vi "SimulatoreStep.vi"() -> ()   [LabVIEW 2019]
doc: "Simulatore Step dei Test:\n\n1. Seleziona la postazione con la data di partenza (opzionale)\n2. Seleziona il Test che vuoi eseguire\n3. Avvia la simulazione e verifica il successo degli Step"
uses:
  ByteGSAPIBase.lvclass
  TypeDef/StepSimulationInfo.ctl
  TypeDef/SimulatoreStates.ctl
  TypeDef/Step.ctl
  TypeDef/Asset.ctl
  TypeDef/Test.ctl
  <vilib>/numeric/Random Number (Range) U64.vi
  <vilib>/numeric/sub_Random U32.vi
panel:
  out "Step Info List":T1[](array[typedef])=[{"info"="Descrizione:\nMeasure T0\nMIN - MAX: 23 - 18", "Value"=0.0, "Outcome"="", "Tempo"=0.0, "id"=0.0}, {"info"="Descrizione:\nSet Nominsl Torque\nMIN - MAX: 1 - -1", "Value"=0.0, "Outcome"="", "Tempo"=0.0, "id"=0.0}, {"info"="Descrizione:\nVibrazione X,Y,Z\nMIN - MAX: 0 - 0", "Value"=0.0, "Outcome"="", "Tempo"=0.0, "id"=0.0}, {"info"="Descrizione:\nPlace Motor on the bench. Plug wires on terminal block.\nMIN - MAX: 0 - 0", "Value"=0.0, "Outcome"="", "Tempo"=0.0, "id"=0.0}, {"info"="Descrizione:\nMeasure R01\nMIN - MAX: 0 - 0", "Value"=0.0, "Outcome"="", "Tempo"=0.0, "id"=0.0}, {"info"="Descrizione:\nMeasure R02\nMIN - MAX: 0 - 0", "Value"=0.0, "Outcome"="", "Tempo"=0.0, "id"=0.0}]
  in  "Step simulation":bool
  out "Infos":string
  in  "Inizia Test":bool
  in  "Seleziona Test":i32(ring) items=["Test Endurance"=36, "Test su Statore H100 dia 65"=31, "Test su Statore H100 dia 65"=29, "Test Endurance"=34, "Test su Statore H100 dia 65"=30, "Effettuare prova sul banco Labview su campione ABC"=40, "Test su Statore H100 dia 65"=28, "Test su Statore H100 dia 65"=32, "Richiesta prova 1"=7, "Test Endurance"=35, "Richiesta prova 1"=5, "Richiesta prova 1"=6, "Test su Statore H100 dia 65"=27, "Test doppio carico per freni 50Nm/12rpm"=24]
  in  "ByteGSAPIBase in":refnum<class "ByteGSAPIBase.lvclass">
  in  "Exit":bool
  in  "Home":bool
  in  "Ottieni Test Per Postazione":bool
  in  "Data Partenza":timestamp format="%<%x>T"
  in  "Postazione":enum16{"POST 1"}(ring)
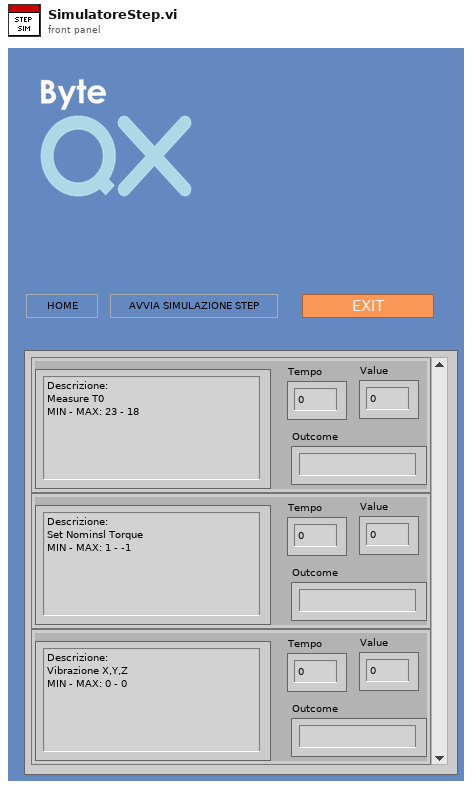
[diagram p1: front panel]
types:
  T1 = typedef "StepSimulationInfo.ctl" = cluster{"info":string, "Value":dbl, "Outcome":string, "Tempo":dbl, "id":dbl}
  T2 = typedef "SimulatoreStates.ctl" = enum16{"Initialize", "Idle", "GetLimsTestsForBench", "GetLimsTestSteps", "Simulation Start"}
  T3 = typedef "ByteGSWebAPI.lvlib/ByteGSAPIBase.lvclass/Test.ctl" = cluster{"titolo":string, "descrizione":string, "statoprova":string, "assets":T4[], "id":i32, "data_apertura_prova":timestamp}
  T4 = typedef "ByteGSWebAPI.lvlib/ByteGSAPIBase.lvclass/Asset.ctl" = cluster{"descrizione":string, "slug":string, "id":i32}
  T5 = typedef "ByteGSWebAPI.lvlib/ByteGSAPIBase.lvclass/Step.ctl" = cluster{"id":i32, "descrizione":string, "prova":string, "assets":T4[], "criterio_accettazione":string, "valore_criterio_accettazione_max":dbl, "valore_criterio_accettazione_min":dbl, "udm_criterio_accettazione":string, "duration_prova":string, "udm_duration_prova":string, "valore_prova":dbl, "outcome":string, "ordine":i32, "user":i32, "link_automation":string, "instruction_automation":string, "data_completamento_checklist":timestamp}
  T6 = cluster{"ByteGSAPIBase in":refnum<class "ByteGSAPIBase.lvclass">, "Array dei Test":T3[], "Steps Array":T5[], "Step Info List":T1[], "index":i32, "Previus":T2, "Infos":string}
  T7 = cluster{"Postazione":refnum<vi>, "Data Partenza":refnum<vi>, "Ottieni Test Per Postazione":refnum<vi>, "Infos":refnum<vi>, "Inizia Test":refnum<vi>, "Seleziona Test":refnum<vi>, "Step Info List":refnum<vi>, "Step simulation":refnum<vi>, "Cluster":refnum<vi>}
  T8 = cluster{"Postazione":enum16{"POST 1"}, "Data Partenza":timestamp, "Seleziona Test":i32}
  T9 = typedef "UpdateLimsTestStepData.ctl" = cluster{"duration_prova":string, "udm_duration_prova":string, "valore_prova":dbl, "outcome":string, "data_completamento_checklist":timestamp, "link_automation":string, "instruction_automation":string}
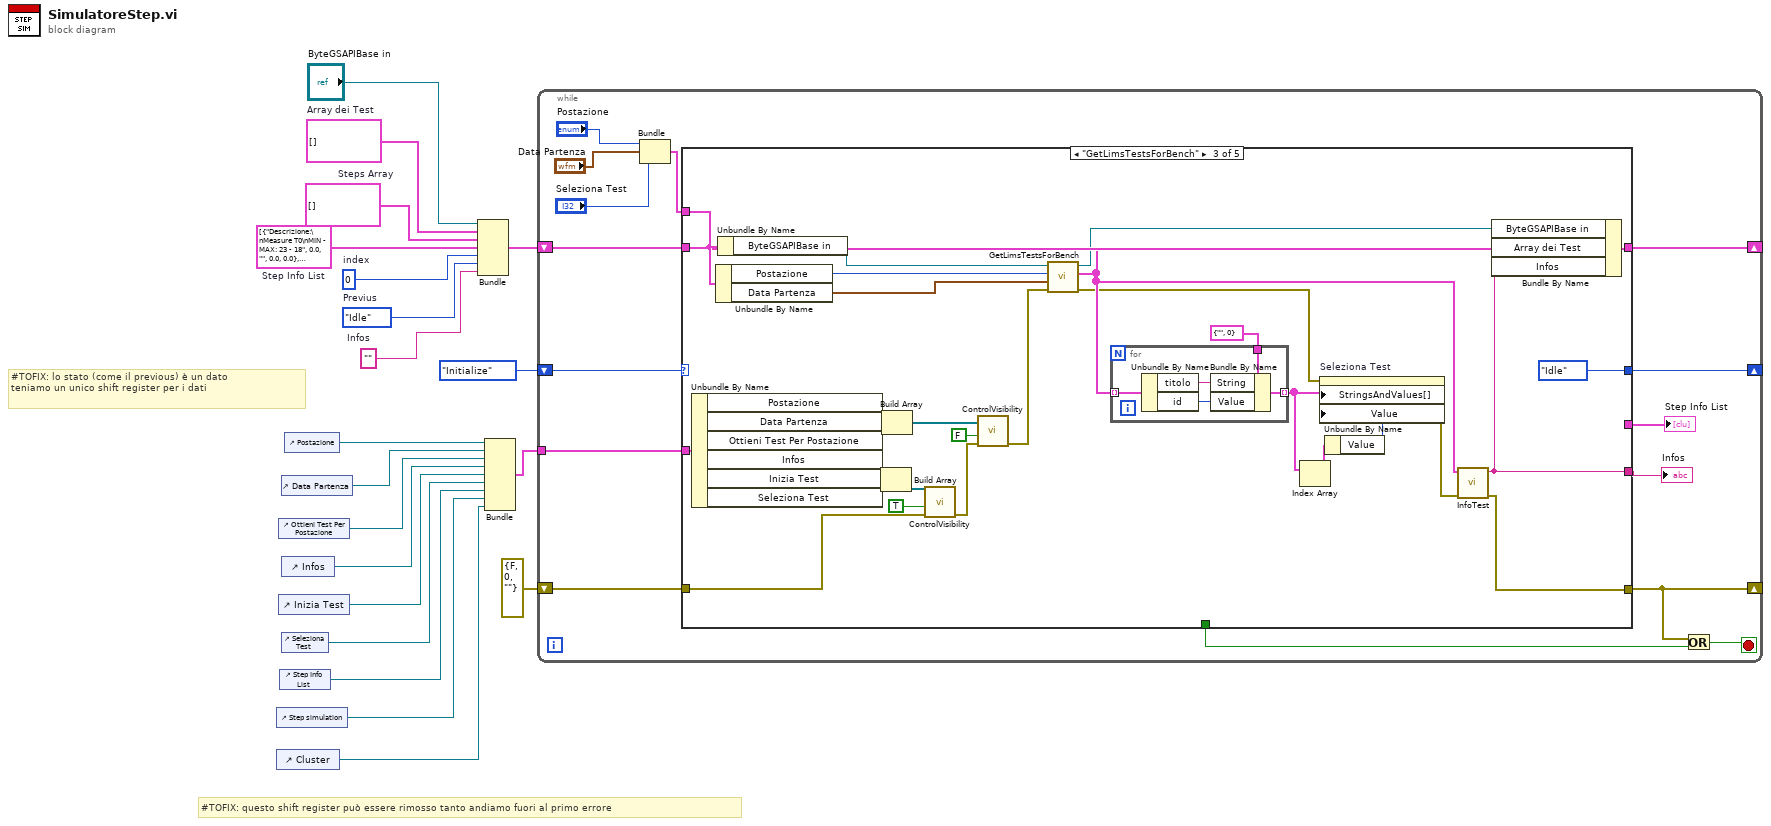
[diagram p0: block diagram]
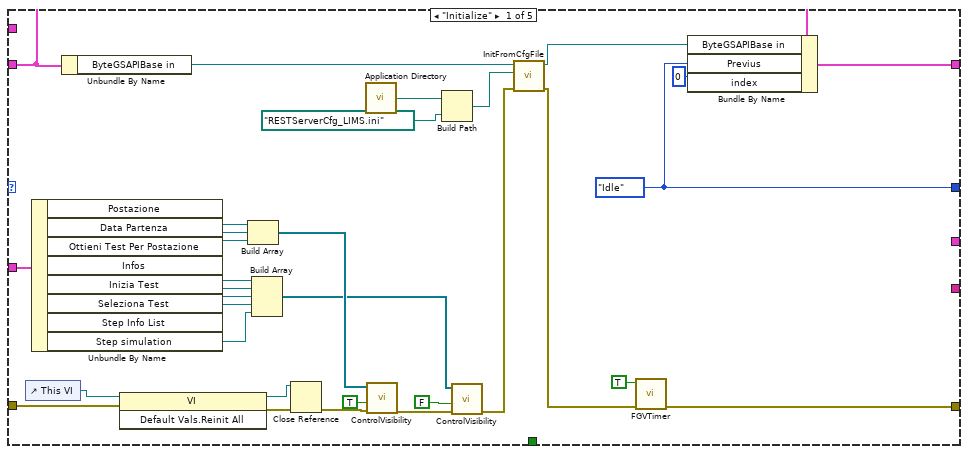
[diagram p2: hidden frame]
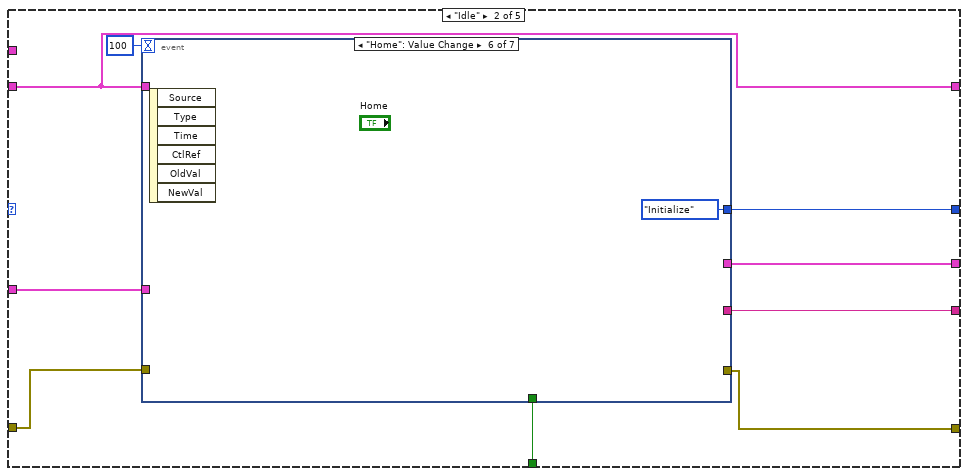
[diagram p3: hidden frame]
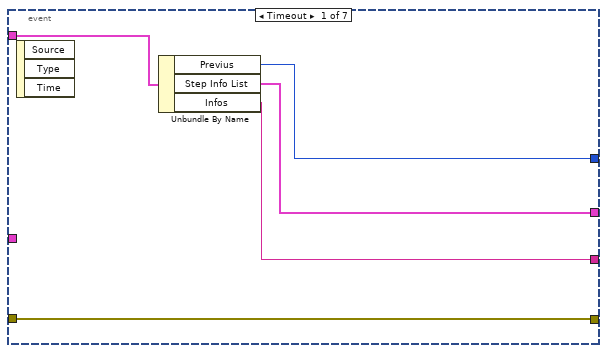
[diagram p4: hidden frame]
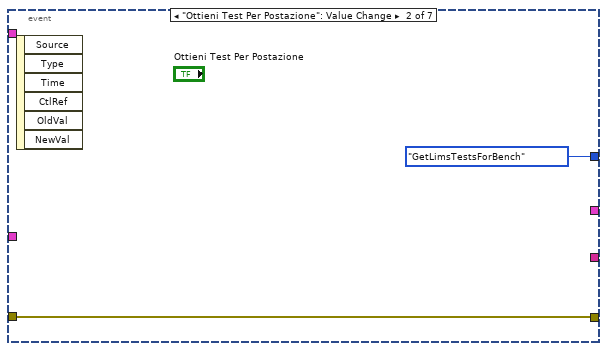
[diagram p5: hidden frame]
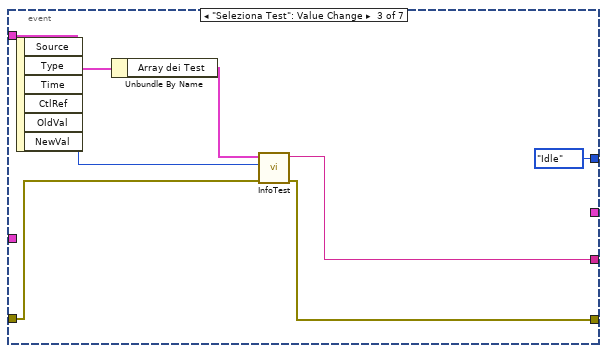
[diagram p6: hidden frame]
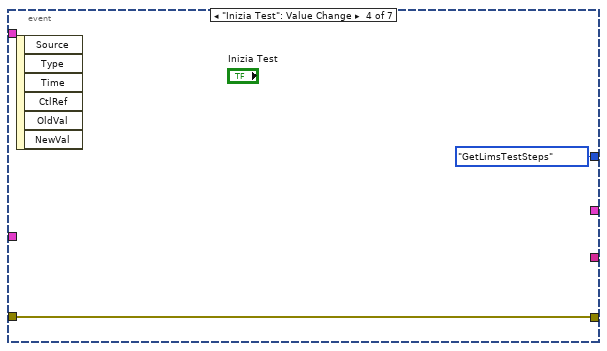
[diagram p7: hidden frame]
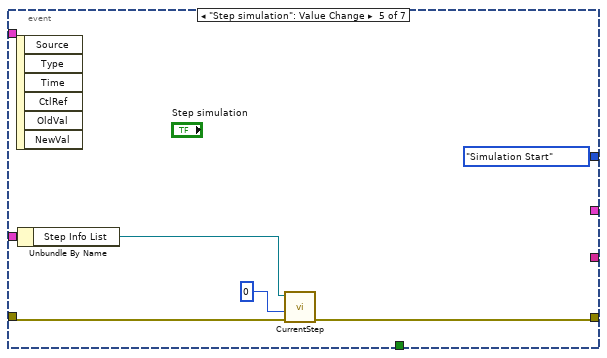
[diagram p8: hidden frame]
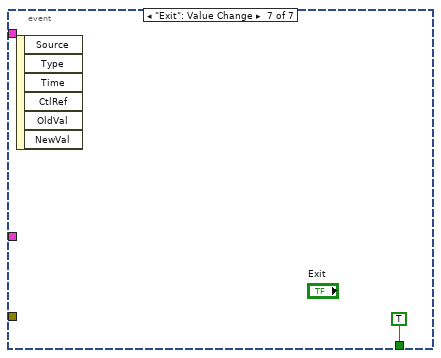
[diagram p9: hidden frame]
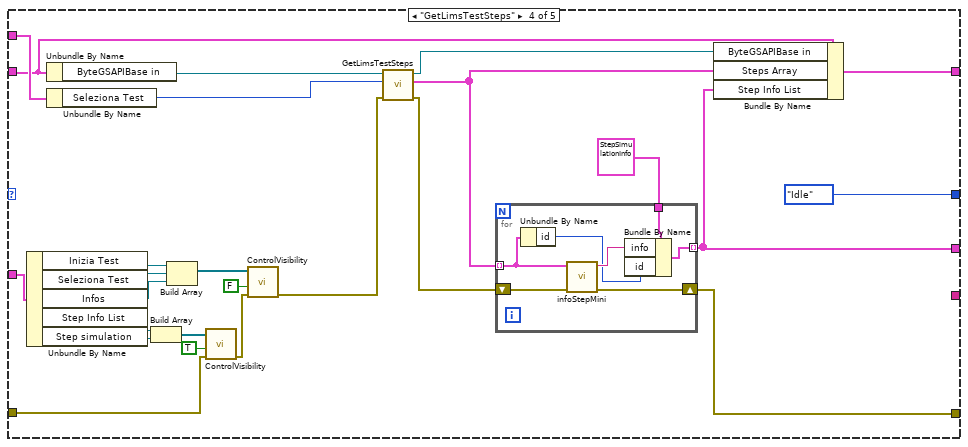
[diagram p10: hidden frame]
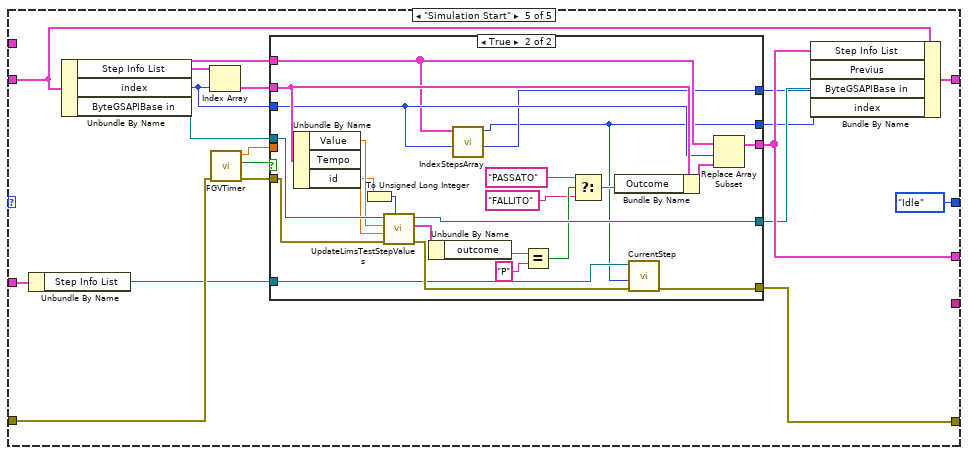
[diagram p11: hidden frame]
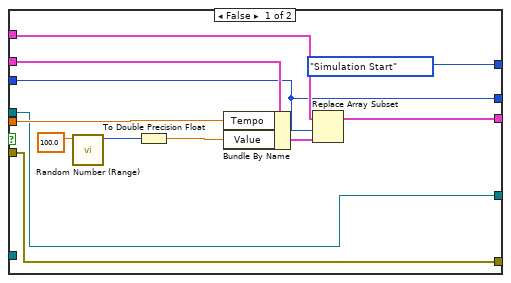
[diagram p12: hidden frame]
diagram:
  w3 = ""  # Infos
  w4 = SimulatoreStates."Idle"  # Previus
  w5 = 0  # index
  w6 = T1[] [{"info"="Descrizione:\nMeasure T0\nMIN - MAX: 23 - 18", "Value"=0.0, "Outcome"="", "Tempo"=0.0, "id"=0.0}, {"info"="Descrizione:\nSet Nominsl Torque\nMIN - MAX: 1 - -1", "Value"=0.0, "Outcome"="", "Tempo"=0.0, "id"=0.0}, {"info"="Descrizione:\nVibrazione X,Y,Z\nMIN - MAX: 0 - 0", "Value"=0.0, "Outcome"="", "Tempo"=0.0, "id"=0.0}, {"info"="Descrizione:\nPlace Motor on the bench. Plug wires on terminal block.\nMIN - MAX: 0 - 0", "Value"=0.0, "Outcome"="", "Tempo"=0.0, "id"=0.0}, {"info"="Descrizione:\nMeasure R01\nMIN - MAX: 0 - 0", "Value"=0.0, "Outcome"="", "Tempo"=0.0, "id"=0.0}, {"info"="Descrizione:\nMeasure R02\nMIN - MAX: 0 - 0", "Value"=0.0, "Outcome"="", "Tempo"=0.0, "id"=0.0}]  # Step Info List
  w13 = T3[] []  # Array dei Test
  w12 = T5[] []  # Steps Array
  # "#TOFIX: questo shift register può essere rimosso tanto andiamo fuori al primo errore"
  # "#TOFIX: lo stato (come il previous) è un dato\nteniamo un unico shift register per i dati"
  n1 = control-ref of="Step simulation"() -> (w7:refnum<vi>)
  n2 = control-ref of="Cluster"() -> (w1:refnum<vi>)
  n3 = control-ref of="Ottieni Test Per Postazione"() -> (w16:refnum<vi>)
  n4 = control-ref of="Inizia Test"() -> (w9:refnum<vi>)
  n5 = control-ref of="Step Info List"() -> (w2:refnum<vi>)
  n6 = control-ref of="Data Partenza"() -> (w17:refnum<vi>)
  n7 = control-ref of="Infos"() -> (w10:refnum<vi>)
  n8 = control-ref of="Seleziona Test"() -> (w8:refnum<vi>)
  n9 = control-ref of="Postazione"() -> (w18:refnum<vi>)
  n10 = Bundle("ByteGSAPIBase in"="ByteGSAPIBase in", "Array dei Test"=w13, "Steps Array"=w12, "Step Info List"=w6, "index"=w5, "Previus"=w4, "Infos"=w3) -> (w11:T6)  [unwired: 1 in]
  n11 = Bundle("Postazione"=w18, "Data Partenza"=w17, "Ottieni Test Per Postazione"=w16, "Infos"=w10, "Inizia Test"=w9, "Seleziona Test"=w8, "Step Info List"=w2, "Step simulation"=w7, "Cluster"=w1) -> (w15:T7)  [unwired: 1 in]
  n12 = while {
    shift-right: [w29] -> _
    shift-left: SimulatoreStates."Initialize" -> [w35]
    shift-right: [w23] -> _
    shift-left: errorcluster {"status"=FALSE, "code"=0, "source"=""} ("error in (no error)") -> [w34]
    tunnel: w15 -> [w30]
    shift-right: [w27] -> _
    shift-left: w11 -> [w28]
    stop <- w22 stop-if-true
    n13 = Bundle("Postazione"="Postazione", "Data Partenza"="Data Partenza", "Seleziona Test"="Seleziona Test") -> (w31:T8)  [unwired: 1 in]
    n14 = case shown="\"GetLimsTestsForBench\"" w35 {
      tunnel: w34 -> [w66 w74 w124 w142 w185]
      tunnel: w31 -> [_ _ w130 w161 _]
      tunnel: w30 -> [w63 w68 w119 w154 w170]
      tunnel: [w39 w73 w108 w147 w173] -> w23
      tunnel: [w38 w76 SimulatoreStates."Idle" SimulatoreStates."Idle" SimulatoreStates."Idle"] -> w29
      tunnel: w28 -> [w51 w72 w129 w158 w182]
      tunnel: [w50 w72 w127 w157 w178] -> w27
      tunnel: [_ w75 w103 _ _] -> w25
      tunnel: [_ w70 _ w138 w179] -> w24
      tunnel: [_ w69 _ _ _] -> w21
      frame "Initialize" {
        w38 = SimulatoreStates."Idle"
        n15 = control-ref of="This VI"() -> (w67:refnum<vi>)
        n16 = Unbundle By Name(w63) -> ("Postazione"=w62:refnum<vi>, "Data Partenza"=w61:refnum<vi>, "Ottieni Test Per Postazione"=w60:refnum<vi>, "Infos"=w46:refnum<vi>, "Inizia Test"=w45:refnum<vi>, "Seleziona Test"=w44:refnum<vi>, "Step Info List"=w42:refnum<vi>, "Step simulation"=w41:refnum<vi>)
        n17 = Unbundle By Name(w51) -> ("ByteGSAPIBase in"=w52:refnum<class "ByteGSAPIBase.lvclass">)
        n18 = invoke class="VI" method="Default Vals.Reinit All"(reference=w67, error in=w66) -> (reference out=w65:refnum<vi>, error out=w64:errorcluster)  [unwired: 1 in, 1 out]
        n19 = Build Array(w62, w61, w60) -> (w59:refnum<vi>[])
        n20 = Build Array(w46, w45, w44, w42, w41) -> (w43:refnum<vi>[])
        n21 = Close Reference(reference=w65, error in (no error)=w64) -> (error out=w58:errorcluster)
        n22 = call <vilib>:"Application Directory.vi"() -> ("Application Directory"=w55:path)
        n23 = call "ControlVisibility.vi"("error in (no error)"=w58, "Visible"=TRUE, "Controls"=w59) -> ("error out"=w49:errorcluster)  [unwired: 8 in]
        n24 = Build Path(base path=w55, name or relative path=path "RESTServerCfg_LIMS.ini") -> (appended path=w56:path)
        n25 = call "ControlVisibility.vi"("error in (no error)"=w49, "Visible"=FALSE, "Controls"=w43) -> ("error out"=w48:errorcluster)  [unwired: 8 in]
        n26 = call-dynamic "InitFromCfgFile.vi"("error in (no error)"=w48, "configuration file path"=w56, "ByteGSAPIBase in"=w52) -> ("error out"=w40:errorcluster, "ByteGSAPIBase out"=w53:refnum<class "ByteGSAPIBase.lvclass">)  [unwired: 7 in]
        n27 = call "FGVTimer.vi"("error in"=w40, "Reset"=TRUE) -> ("error out"=w39:errorcluster)  [unwired: 7 in, 2 out]
        n28 = Bundle By Name(cluster=w51, "ByteGSAPIBase in"=w53, "Previus"=w38, "index"=0) -> (w50:T6)
      }
      frame "Idle" {
        n29 = event shown="[5] \"Home\": Value Change" {
          selector: _ -> [_ _ _ _ _ _ _]
          dyn-events: _ -> [_ _ _ _ _ _ _]
          timeout: 100 -> [_ _ _ _ _ _ _]
          tunnel: [w80 SimulatoreStates."GetLimsTestsForBench" SimulatoreStates."Idle" SimulatoreStates."GetLimsTestSteps" SimulatoreStates."Simulation Start" SimulatoreStates."Initialize" _] -> w76
          tunnel: [w78 _ w88 _ _ _ _] -> w75
          tunnel: w74 -> [w77 w82 w87 w91 w96 _ _]
          tunnel: [w77 w82 w86 w91 w95 _ _] -> w73
          tunnel: w72 -> [w81 _ w85 _ _ _ _]
          tunnel: [w79 _ _ _ _ _ _] -> w70
          tunnel: [_ _ _ _ _ _ TRUE] -> w69
          tunnel: w68 -> [_ _ _ _ w97 _ _]
          event Timeout {
            n30 = event-data() -> ()  [unwired: 1 in, 3 out]
            n31 = Unbundle By Name(w81) -> ("Previus"=w80:T2, "Step Info List"=w79:T1[], "Infos"=w78:string)
          }
          event "Ottieni Test Per Postazione": Value Change {
            n32 = event-data() -> ()  [unwired: 1 in, 6 out]
          }
          event "Seleziona Test": Value Change {
            n33 = event-data() -> ("NewVal"=w84:i32)  [unwired: 1 in, 5 out]
            n34 = Unbundle By Name(w85) -> ("Array dei Test"=w89:T3[])
            n35 = call "InfoTest.vi"("error in"=w87, "Seleziona Test"=w84, "TestForBenchArray"=w89) -> ("error out"=w86:errorcluster, "Info Test"=w88:string)  [unwired: 7 in]
          }
          event "Inizia Test": Value Change {
            n36 = event-data() -> ()  [unwired: 1 in, 6 out]
          }
          event "Step simulation": Value Change {
            n37 = event-data() -> ()  [unwired: 1 in, 6 out]
            n38 = Unbundle By Name(w97) -> ("Step Info List"=w94:refnum<vi>)
            n39 = call "CurrentStep.vi"("error in (no error)"=w96, "index"=0, "Array in"=w94) -> ("error out"=w95:errorcluster)  [unwired: 8 in]
          }
          event "Home": Value Change {
            n40 = event-data() -> ()  [unwired: 1 in, 6 out]
          }
          event "Exit": Value Change {
            n41 = event-data() -> ()  [unwired: 1 in, 6 out]
          }
        }
      }
      frame "GetLimsTestsForBench" {
        n42 = Unbundle By Name(w119) -> ("Postazione"=w118:refnum<vi>, "Data Partenza"=w117:refnum<vi>, "Ottieni Test Per Postazione"=w116:refnum<vi>, "Infos"=w115:refnum<vi>, "Inizia Test"=w114:refnum<vi>, "Seleziona Test"=w113:refnum<vi>)
        n43 = Unbundle By Name(w130) -> ("Postazione"=w102:enum16{"POST 1"}, "Data Partenza"=w101:timestamp)
        n44 = Unbundle By Name(w129) -> ("ByteGSAPIBase in"=w131:refnum<class "ByteGSAPIBase.lvclass">)
        n45 = Build Array(w115, w114, w113) -> (w106:refnum<vi>[])
        n46 = Build Array(w118, w117, w116) -> (w107:refnum<vi>[])
        n47 = call "ControlVisibility.vi"("error in (no error)"=w124, "Visible"=TRUE, "Controls"=w106) -> ("error out"=w112:errorcluster)  [unwired: 8 in]
        n48 = call "ControlVisibility.vi"("error in (no error)"=w112, "Visible"=FALSE, "Controls"=w107) -> ("error out"=w111:errorcluster)  [unwired: 8 in]
        n49 = call-dynamic "GetLimsTestsForBench.vi"("error in (no error)"=w111, "Data Partenza"=w101, "Postazione"=w102, "ByteGSAPIBase in"=w131) -> ("error out"=w110:errorcluster, "Tests for bench"=w120:T3[], "ByteGSAPIBase out"=w128:refnum<class "ByteGSAPIBase.lvclass">)  [unwired: 5 in]
        n50 = for {
          tunnel: w120 -> [w136] mode=indexing
          tunnel: [w133] -> w123 mode=indexing
          tunnel: cluster{"String":string, "Value":u16} {"String"="", "Value"=0} ("Cluster") -> [w132]
          n51 = Unbundle By Name(w136) -> ("titolo"=w135:string, "id"=w134:i32)
          n52 = Bundle By Name(cluster=w132, "String"=w135, "Value"=w134) -> (w133:cluster{"String":string, "Value":u16})
        }
        n53 = Index Array(array=w123) -> (element=w122:cluster{"String":string, "Value":u16})  [unwired: 1 in]
        n54 = Unbundle By Name(w122) -> ("Value"=w121:u16)
        n55 = property on="Seleziona Test" class="Ring (strict)"(error in=w110, "StringsAndValues[]"=w123, "Value"=w121) -> (error out=w109:errorcluster)  [unwired: 1 in, 1 out]
        n56 = call "InfoTest.vi"("error in"=w109, "TestForBenchArray"=w120) -> ("error out"=w108:errorcluster, "Info Test"=w103:string)  [unwired: 8 in]
        n57 = Bundle By Name(cluster=w129, "ByteGSAPIBase in"=w128, "Array dei Test"=w120, "Infos"=w103) -> (w127:T6)
      }
      frame "GetLimsTestSteps" {
        n58 = Unbundle By Name(w154) -> ("Inizia Test"=w153:refnum<vi>, "Seleziona Test"=w152:refnum<vi>, "Infos"=w145:refnum<vi>, "Step Info List"=w144:refnum<vi>, "Step simulation"=w139:refnum<vi>)
        n59 = Unbundle By Name(w158) -> ("ByteGSAPIBase in"=w160:refnum<class "ByteGSAPIBase.lvclass">)
        n60 = Unbundle By Name(w161) -> ("Seleziona Test"=w146:i32)
        n61 = Build Array(w144, w139) -> (w143:refnum<vi>[])
        n62 = Build Array(w153, w152, w145) -> (w151:refnum<vi>[])
        n63 = call "ControlVisibility.vi"("error in (no error)"=w142, "Visible"=TRUE, "Controls"=w143) -> ("error out"=w141:errorcluster)  [unwired: 8 in]
        n64 = call "ControlVisibility.vi"("error in (no error)"=w141, "Visible"=FALSE, "Controls"=w151) -> ("error out"=w150:errorcluster)  [unwired: 8 in]
        n65 = call-dynamic "GetLimsTestSteps.vi"("error in (no error)"=w150, "Test-id"=w146, "ByteGSAPIBase in"=w160) -> ("error out"=w148:errorcluster, "Test Steps List"=w149:T5[], "ByteGSAPIBase out"=w159:refnum<class "ByteGSAPIBase.lvclass">)  [unwired: 6 in]
        n66 = for {
          tunnel: w149 -> [w163] mode=indexing
          shift-right: [w167] -> w147
          shift-left: w148 -> [w168]
          tunnel: T1 {"info"="Descrizione:\nMeasure T0\nMIN - MAX: 23 - 18", "Value"=0.0, "Outcome"="", "Tempo"=0.0, "id"=0.0} ("Cluster") -> [w166]
          tunnel: [w164] -> w138 mode=indexing
          n67 = Unbundle By Name(w163) -> ("id"=w162:i32)
          n68 = call "infoStepMini.vi"("error in (no error)"=w168, "StepList"=w163) -> ("error out"=w167:errorcluster, "Info Test"=w165:string)  [unwired: 8 in]
          n69 = Bundle By Name(cluster=w166, "info"=w165, "id"=w162) -> (w164:T1)
        }
        n70 = Bundle By Name(cluster=w158, "ByteGSAPIBase in"=w159, "Steps Array"=w149, "Step Info List"=w138) -> (w157:T6)
      }
      frame "Simulation Start" {
        n71 = Unbundle By Name(w170) -> ("Step Info List"=w169:refnum<vi>)
        n72 = Unbundle By Name(w182) -> ("Step Info List"=w181:T1[], "index"=w180:i32, "ByteGSAPIBase in"=w176:refnum<class "ByteGSAPIBase.lvclass">)
        n73 = Index Array(array=w181, index=w180) -> (element=w184:T1)
        n74 = call "FGVTimer.vi"("error in"=w185) -> ("error out"=w175:errorcluster, "Elapsed?"=w186:bool, "Time Elapsed"=w183:dbl)  [unwired: 8 in]
        n75 = case shown="True" w186 {
          tunnel: w184 -> [w198 w218]
          tunnel: w183 -> [w196 _]
          tunnel: w181 -> [w195 w210]
          tunnel: w180 -> [w187 w211]
          tunnel: [w193 w222] -> w179
          tunnel: w176 -> [w192 w220]
          tunnel: w175 -> [w188 w219]
          tunnel: [w192 w213] -> w174
          tunnel: [w188 w202] -> w173
          tunnel: [w187 w199] -> w172
          tunnel: [SimulatoreStates."Simulation Start" ("Previus") w209] -> w171
          tunnel: w169 -> [_ w200]
          frame False {
            n76 = call-poly <vilib>:"Random Number (Range).vi"("upper bound (100)"=100.0) -> ("number"=w190:u64)  [unwired: 10 in]
            n77 = To Double Precision Float(number=w190) -> (double precision float=w189:dbl)
            n78 = Bundle By Name(cluster=w198, "Tempo"=w196, "Value"=w189) -> (w194:T1)
            n79 = Replace Array Subset(array=w195, new element=w194, index=w187) -> (w193:T1[])
          }
          frame True {
            n80 = Unbundle By Name(w218) -> ("Value"=w217:dbl, "Tempo"=w216:dbl, "id"=w214:dbl)
            n81 = To Unsigned Long Integer(number=w214) -> (unsigned 32bit integer=w215:u32)
            n82 = call-dynamic "UpdateLimsTestStepValues.vi"("step_id"=w215, "error in (no error)"=w219, "duration_hours"=w216, "value"=w217, "ByteGSAPIBase in"=w220) -> ("error out"=w201:errorcluster, "Result Step"=w212:T9, "ByteGSAPIBase out"=w213:refnum<class "ByteGSAPIBase.lvclass">)  [unwired: 4 in]
            n83 = Unbundle By Name(w212) -> ("outcome"=w207:string)
            n84 = call "IndexStepsArray.vi"("index"=w211, "Steps Array"=w210) -> ("Previus"=w209:T2, "Index out"=w199:i32)  [unwired: 8 in]
            n85 = Equal?(x=w207, y="P") -> (x = y?=w205:bool)
            n86 = Select(t="PASSATO", s=w205, f="FALLITO") -> (s? t:f=w208:string)
            n87 = Bundle By Name(cluster=w218, "Outcome"=w208) -> (w221:T1)
            n88 = call "CurrentStep.vi"("error in (no error)"=w201, "index"=w199, "Array in"=w200) -> ("error out"=w202:errorcluster)  [unwired: 8 in]
            n89 = Replace Array Subset(array=w210, new element=w221, index=w211) -> (w222:T1[])
          }
        }
        n90 = Bundle By Name(cluster=w182, "Step Info List"=w179, "Previus"=w171, "ByteGSAPIBase in"=w174, "index"=w172) -> (w178:T6)
      }
    }
    "Infos" <- w25
    "Step Info List" <- w24
    n91 = Or(x=w23, y=w21) -> (x .or. y?=w22:bool)
  }
